vi "FIFOEmpty.vi"(0 "FPGA VI Reference In":T1, 1 "error in (no error)":errorcluster) -> (7 "FPGA VI Reference Out":T1, 8 "error out":errorcluster, 9 "RX_EMPTY":bool)   [LabVIEW 2016]
uses:
  FPGA Bitfiles/FPGA_defref.ctl
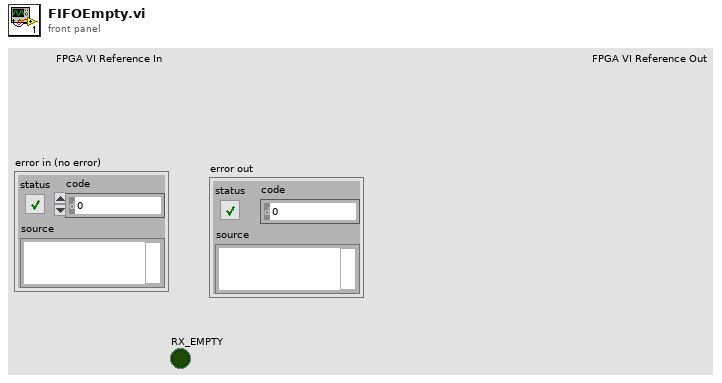
[diagram p1: front panel]
types:
  T1 = typedef "FPGA_defref.ctl" = refnum<k20>
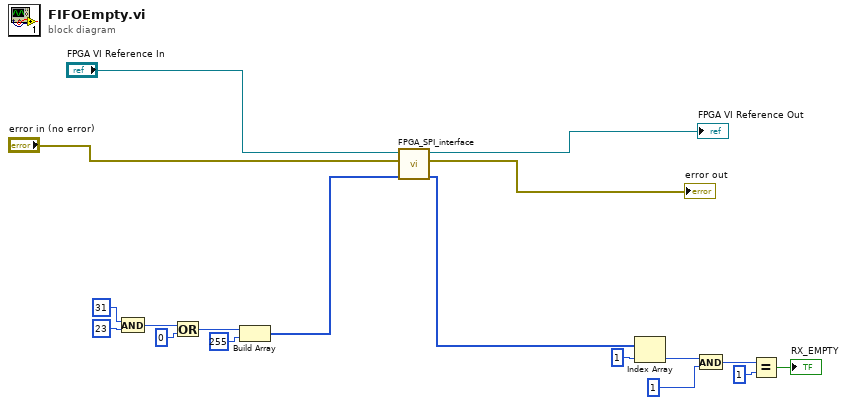
[diagram p0: block diagram]
diagram:
  n1 = And(x=31, y=23) -> (x .and. y?=w9:i32)
  n2 = Or(x=w9, y=0) -> (x .or. y?=w7:i32)
  n3 = Build Array(w7, 255) -> (w6:i32[])
  n4 = call "FPGA_SPI_interface.vi"("Frames to Write"=w6, "error in"="error in (no error)", "FPGA VI Reference In"="FPGA VI Reference In") -> ("Frames Read"=w5:u8[], "error out"=→"error out":errorcluster, "FPGA VI Reference Out"=→"FPGA VI Reference Out":T1)  [unwired: 6 in]
  n5 = Index Array(array=w5, index=1) -> (element=w14:u8)
  n6 = And(x=w14, y=u8 1) -> (x .and. y?=w16:u8)
  n7 = Equal?(x=w16, y=u8 1) -> (x = y?=→"RX_EMPTY":bool)
